vi "LabVLC - VolumeControl.vi"(2 "error in (no error)":errorcluster, 3 "volume (percents)":i32(knob) min=0 max=100 step=1 scale=0.0..100.0, 4 "struct":T1={"media_ptr"=0, "vlc_inst_ptr"=0, "path in"=path "C:/Program Files (x86)/VideoLAN/VLC/libvlc.dll"}) -> (0 "error out":errorcluster, 1 "out":T1)   [LabVIEW 2014]
doc: "Controls VLC playback volume. 100 is default. Numbers are percentages of overall volume. You may mute the video by setting volume to zero, or you may use the mute function. 32 bit integer for the input only. Requires a media pointer. Mute function call overrides volume control.s"
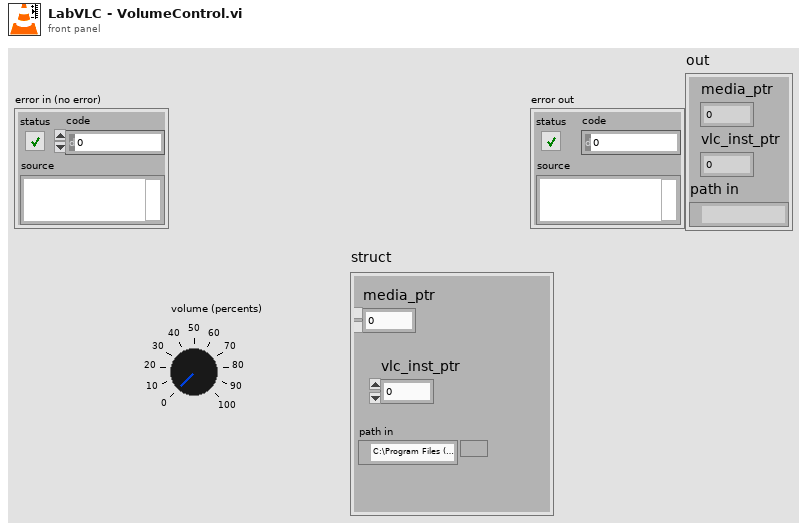
[diagram p1: front panel]
types:
  T1 = cluster{"media_ptr":i32, "vlc_inst_ptr":i32, "path in":path}
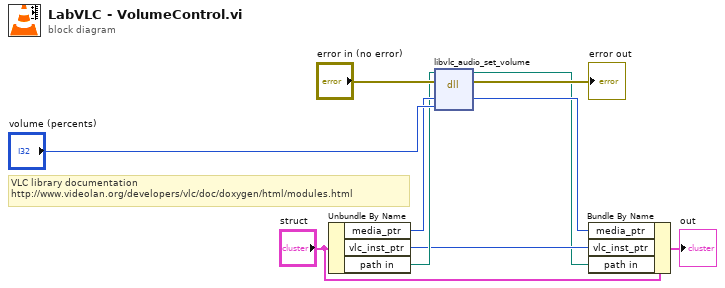
[diagram p0: block diagram]
diagram:
  # "VLC library documentation\nhttp://www.videolan.org/developers/vlc/doc/doxygen/html/modules.html"
  n1 = Unbundle By Name("struct") -> ("media_ptr"=w6:i32, "vlc_inst_ptr"=w4:i32, "path in"=w5:path)
  n2 = dll-call lib="C:/Program Files (x86)/VideoLAN/VLC/libvlc.dll" fn="libvlc_audio_set_volume"(path in=w5, error in="error in (no error)", "media_pointer"=w6, "volume (percents)"="volume (percents)") -> (path out=w2:path, error out=→"error out":errorcluster, "media_pointer"=w3:i32)  [unwired: 3 in]
  n3 = Bundle By Name(cluster="struct", "media_ptr"=w3, "vlc_inst_ptr"=w4, "path in"=w2) -> (→"out":T1)
